vi "LabvolutionSubmoduleCheck_FindFolders.vi"(11 "Project Dir":path) -> (3 "Folders":path[](array[path]))   [LabVIEW 2018]
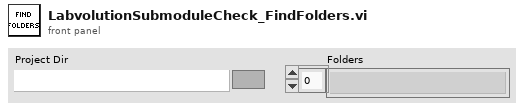
[diagram p1: front panel]
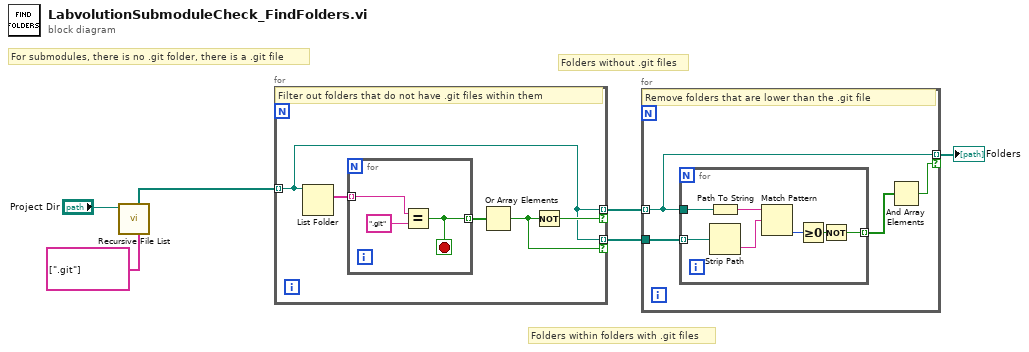
[diagram p0: block diagram]
diagram:
  # "Folders within folders with .git files"
  # "Folders without .git files"
  # "For submodules, there is no .git folder, there is a .git file"
  n1 = call <vilib>:"Recursive File List.vi"("Folders to Exclude"=string[] [".git"], "Folder Path"="Project Dir") -> ("All Folders"=w4:path[])  [unwired: 5 in, 4 out]
  n2 = for {
    tunnel: w4 -> [w8] mode=indexing
    tunnel: [w8] -> w3 mode=indexing if=w9
    tunnel: [w8] -> w2 mode=indexing if=w7
    # "Filter out folders that do not have .git files within them"
    n3 = List Folder(path=w8) -> (filenames=w11:string[])  [unwired: 3 in, 3 out]
    n4 = for {
      tunnel: w11 -> [w14] mode=indexing
      tunnel: [w12] -> w10 mode=indexing
      stop <- w12 stop-if-true
      n5 = Equal?(x=w14, y=".git") -> (x = y?=w12:bool)
    }
    n6 = Or Array Elements(Boolean array=w10) -> (logical OR=w7:bool)
    n7 = Not(x=w7) -> (.not. x?=w9:bool)
  }
  n8 = for {
    tunnel: w3 -> [w15] mode=indexing
    tunnel: w2 -> [w18]
    tunnel: [w15] -> w1 mode=indexing if=w16
    # "Remove folders that are lower than the .git file"
    n9 = for {
      tunnel: w18 -> [w20] mode=indexing
      tunnel: w15 -> [w23]
      tunnel: [w21] -> w17 mode=indexing
      n10 = Path To String(path=w23) -> (string=w25:string)
      n11 = Strip Path(path=w20) -> (name=w19:string)  [unwired: 1 out]
      n12 = Match Pattern(string=w25, regular expression=w19) -> (offset past match=w24:i32)  [unwired: 1 in, 3 out]
      n13 = Greater Or Equal To 0?(x=w24) -> (x >= 0?=w22:bool)
      n14 = Not(x=w22) -> (.not. x?=w21:bool)
    }
    n15 = And Array Elements(Boolean array=w17) -> (logical AND=w16:bool)
  }
  "Folders" <- w1
